vi "XYZStage-Read speed setting command.vi"(8 "error in (no error)":errorcluster, 9 "XYZ Stage data to queue":T1={"Command"=enum."Initialize", "Channel"="Z", "X"=0.0, "Y"=0.0, "Z"=0.0, "Speed"=0, "Zero"=FALSE, "Use acknowledgement?"=TRUE} {"Speed" format="Speed= %.0f"; "Z" format="Z= %#_g"; "Y" format="Y= %#_g"; "X" format="X= %#_g"}, 10 "XY Stage config cluster":T4) -> (0 "error out":errorcluster)   [LabVIEW 2013]
doc: "Reads the XYZ Stage coordinates"
uses:
  Typedefs/XY Stage config cluster.ctl
  Typedefs/XYZ stage data.ctl
  Typedefs/XYZ stage states.ctl
  Typedefs/XYZ channel ring.ctl
  Typedefs/Command acknowledgment states.ctl
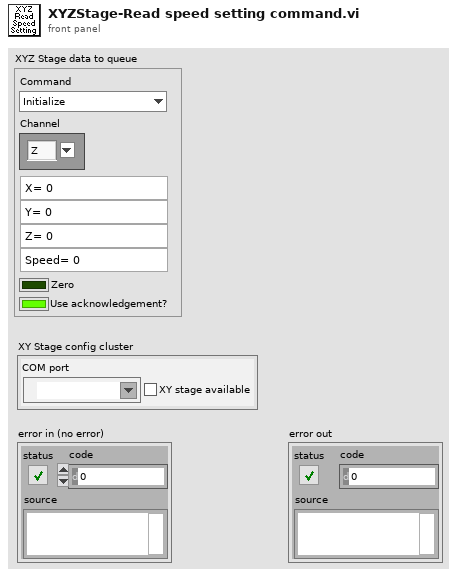
[diagram p1: front panel]
types:
  T1 = typedef "XYZ stage data.ctl" = cluster{"Command":T2, "Channel":T3, "X":sgl, "Y":sgl, "Z":sgl, "Speed":i32, "Zero":bool, "Use acknowledgement?":bool}
  T2 = typedef "XYZ stage states.ctl" = enum16{"Dequeue", "Initialize", "Read Position", "Read Speed Setting", "Move", "Set Max Speed", "Reset Axis", "Stop all movement"}
  T3 = typedef "XYZ channel ring.ctl" = string
  T4 = typedef "XY Stage config cluster.ctl" = cluster{"COM port":refnum<visa-resource-name>, "XY stage available":bool}
  T5 = typedef "Command acknowledgment states.ctl" = enum16{"Acknowledge", "Wait for acknowledgment", "Release queue"}
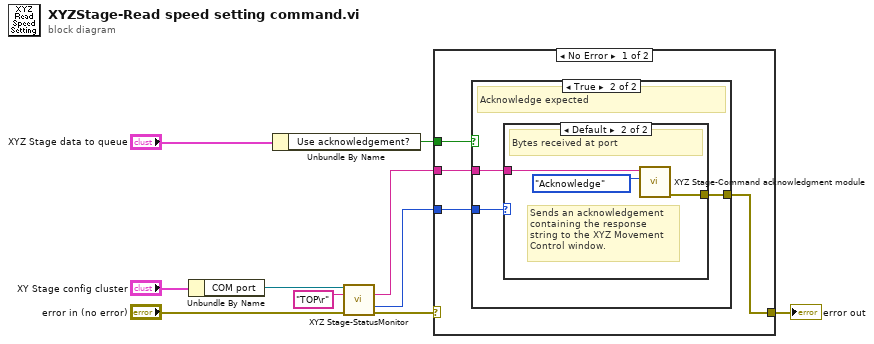
[diagram p0: block diagram]
diagram:
  n1 = Unbundle By Name("XY Stage config cluster") -> ("COM port"=w8:refnum<visa-resource-name>)
  n2 = Unbundle By Name("XYZ Stage data to queue") -> ("Use acknowledgement?"=w7:bool)
  n3 = call "XYZ Stage-StatusMonitor.vi"("VISA resource name"=w8, "string to write"="TOP\r", "Error In"="error in (no error)") -> ("read string"=w4:string, "bytes read"=w1:u32, "Error Out"=w3:errorcluster)  [unwired: 8 in, 2 out]
  n4 = case shown="No Error" w3 {
    selector: w3 -> [_ w21]
    tunnel: w7 -> [w14 _]
    tunnel: w4 -> [w13 _]
    tunnel: [w12 w21] -> w2
    tunnel: w1 -> [w11 _]
    frame No Error {
      n5 = case shown="True" w14 {
        tunnel: w13 -> [_ w17]
        tunnel: [_ w16] -> w12
        tunnel: w11 -> [_ w15]
        frame False {
          # "No acknowledgement expected"
        }
        frame True {
          # "Acknowledge expected"
          n6 = case shown="Default" w15 {
            tunnel: w17 -> [_ w19]
            tunnel: [_ w18] -> w16
            frame 0 {
              # "No data at port"
            }
            frame Default {
              # "Sends an acknowledgement containing the response string to the XYZ Movement Control window."
              # "Bytes received at port"
              n7 = call "XYZ Stage-Command acknowledgment module.vi"("State"=Command_acknowledgment_states."Acknowledge", "Acknowledgement Message in"=w19) -> ("error out"=w18:errorcluster)  [unwired: 7 in, 2 out]
            }
          }
        }
      }
    }
    frame Error {
    }
  }
  "error out" <- w2
